vi "find_calibration.vi"(10 "Calibration in":T1 {"r bias" format="%_3p"; "Ks" format="%#_3p"}, 11 "Cal data":dbl[][](array[numeric])) -> (1 "f(minimum)":dbl, 2 "Calibration out":T1 {"r bias" format="%_3p"; "Ks" format="%#_3p"}, 3 "Residuals":dbl[](array[numeric]), 4 "status":bool)   [LabVIEW 2026]
uses:
  calibration.ctl
  <vilib>/gmath/NumericalOptimization/stopping criteria.ctl
  <vilib>/gmath/NumericalOptimization/Downhill Simplex.vi
  <vilib>/gmath/NI_Gmath.lvlib
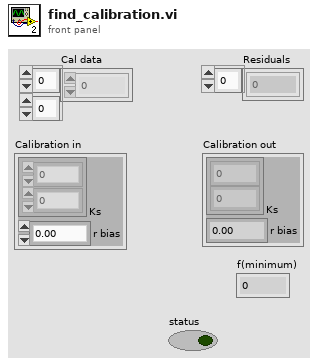
[diagram p1: front panel]
types:
  T1 = typedef "calibration.ctl" = cluster{"Ks":dbl[], "r bias":dbl}
  T2 = typedef "NI_Gmath.lvlib/stopping criteria.ctl" = cluster{"function tolerance":dbl, "parameter tolerance":dbl, "max iterations":i32, "max function calls":i32, "gradient tolerance":dbl, "max time (sec)":dbl}
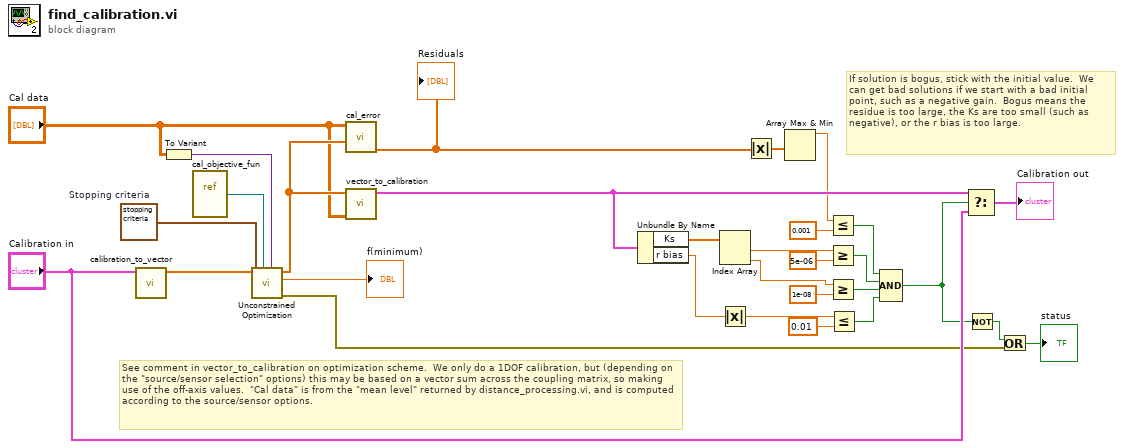
[diagram p0: block diagram]
diagram:
  w28 = T2 {"function tolerance"=1e-06, "parameter tolerance"=1e-06, "max iterations"=1000, "max function calls"=2000, "gradient tolerance"=1e-06, "max time (sec)"=-1.0}  # Stopping criteria
  # "If solution is bogus, stick with the initial value.  We can get bad solutions if we start with a bad initial point, such as a negative gain.  Bogus means the residue is too large, the Ks are too small (such as negative), or the r bias is too large."
  # "See comment in vector_to_calibration on optimization scheme.  We only do a 1DOF calibration, but (depending on the \"source/sensor selection\" options) this may be based on a vector sum across the coupling matrix, so making use of the off-axis values.  \"Cal data\" is from the \"mean level\" returned by distance_processing.vi, and is computed according to the source/sensor options."
  n1 = call "calibration_to_vector.vi"("Calibration in"="Calibration in") -> ("State vector"=w30:dbl[])  [unwired: 10 in]
  n2 = To Variant(anything="Cal data") -> (Variant=w26:variant)
  n3 = vi-ref "cal_objective_fun.vi"() -> (w27:refnum<vi>)
  n4 = call-poly <vilib>:"Unconstrained Optimization.vi"("function data"=w26, "objective function"=w27, "stopping criteria"=w28, "start"=w30) -> ("error out"=w10:errorcluster, "f(minimum)"=→"f(minimum)":dbl, "minimum"=w29:dbl[])  [unwired: 1 in, 4 out]
  n5 = call "cal_error.vi"("X"=w29, "Cal data"="Cal data") -> ("Residuals"=w7:dbl[])  [unwired: 8 in, 1 out]
  "Residuals" <- w7
  n6 = call "vector_to_calibration.vi"("Cal data"="Cal data", "minimum"=w29) -> ("Calibration out"=w13:T1)  [unwired: 9 in]
  n7 = Unbundle By Name(w13) -> ("Ks"=w2:dbl[], "r bias"=w19:dbl)
  n8 = Index Array(array=w2) -> (element #1=w23:dbl, element #2=w20:dbl)  [unwired: 2 in]
  n9 = Absolute Value(x=w19) -> (abs(x)=w18:dbl)
  n10 = Absolute Value(x=w7) -> (abs(x)=w6:dbl[])
  n11 = Array Max & Min(array=w6) -> (max value=w4:dbl)  [unwired: 3 out]
  n12 = Less Or Equal?(x=w4, y=0.001) -> (x <= y?=w3:bool)
  n13 = Greater Or Equal?(x=w23, y=5e-06) -> (x >= y?=w16:bool)
  n14 = Greater Or Equal?(x=w20, y=1e-08) -> (x >= y?=w15:bool)
  n15 = Less Or Equal?(x=w18, y=0.01) -> (x <= y?=w14:bool)
  n16 = Compound Arithmetic op=AND(w3, w16, w15, w14) -> (w1:bool)
  n17 = Select(t=w13, s=w1, f="Calibration in") -> (s? t:f=→"Calibration out":T1)
  n18 = Not(x=w1) -> (.not. x?=w9:bool)
  n19 = Or(x=w9, y=w10) -> (x .or. y?=→"status":bool)
